vi "SSH_Write.vi"(8 "error in (no error)":errorcluster, 10 "Text to write":string, 11 "Python in":cluster{"Python":refnum<k35>, "py file":path}) -> (0 "error out":errorcluster, 3 "Python out":cluster{"Python":refnum<k35>, "py file":path})   [LabVIEW 2020]
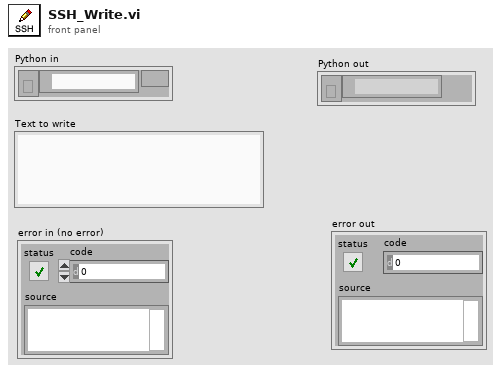
[diagram p1: front panel]
types:
  T1 = cluster{"session out":refnum<k35>, "py file":path}
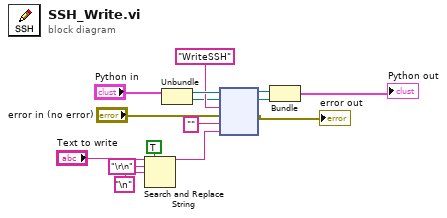
[diagram p0: block diagram]
diagram:
  n1 = Search and Replace String(replace all?=TRUE ("replace all? (F)"), input string="Text to write", search string="\r\n", replace string="\n" ("search string")) -> (result string=w12:string)  [unwired: 4 in, 3 out]
  n2 = Unbundle("Python in") -> ("Python"=w13:refnum<k35>, "py file"=w2:path)
  n3 = node(w13, w2, "WriteSSH" ("function name"), "error in (no error)", "" ("function name"), w12) -> (w3:refnum<k35>, →"error out":errorcluster)  [unwired: 2 in, 2 out]
  n4 = Bundle("session out"=w3, "py file"=w2) -> (→"Python out":T1)  [unwired: 1 in]
